vi "PH_Synchrolock_Watch.destructor.vi"(0 "i ref in":refnum<vi>, 5 "error in(no error)":errorcluster) -> (19 "error out":errorcluster)   [LabVIEW 2014, in "PH_Synchrolock_Watch.lvlib"]
doc: "This is the destructor of a class.\n\nLicense Agreement for this software:\n\nCopyright (C)\nGesellschaft für Schwerionenforschung, GSI\nPlanckstr. 1\n64291 Darmstadt\nGermany\n\nContact: D.Beck@gsi.de \n\nThis program is free software; you can redistribute it and/or modify it under the terms of the \nGNU General Public License as published by the Free Software Foundation; either version 2 of \nthe license, or (at your option) any later version.\n\nThis program is distributed in the hope that it will be useful, but WITHOUT ANY WARRANTY; \nwithout even the implied warranty of MERCHANTABILITY or FITNESS FOR A PARTICULAR PURPOSE. See the GNU General License for more details (http://www.gnu.org).\n\nGesellschaft für Schwerionenforschung, GSI\nPlanckstr. 1, 64291 Darmstadt, Germany\nFor all questions and ideas contact: M.Richter@gsi.de, H.Brand@gsi.de or D.Beck@gsi.de.\nLast update: 16-JUN-2004"
uses:
  PH_Synchrolock_Watch.lvlib
  PH_Devices/PH_TKTDS-30xx/PH_TKTDS-30xx.lvlib
  CS_Core/BaseProcess/BaseProcess.lvlib
  PH_Basics/PH_StatusHandler/PH_StatusHandler.lvlib
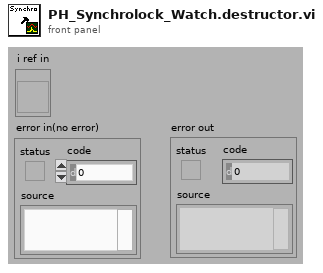
[diagram p1: front panel]
types:
  T1 = typedef "BaseProcess.lvlib/BaseProcess.i attribute.ctl" = cluster{"EventStatus":string, "EventError":i32, "PresetEvtWatchD":i32, "PresetPdcWatchD":i32, "EventTimeout":i32, "PeriodicInterval":i32, "Interface":string[], "Address":string[], "Special":string[], "PeriodicError":i32, "PeriodicStatus":string, "SuperProc":string, "Descriptors":T2[], "CaseRef":refnum<vi>, "PdcRef":refnum<vi>, "Thread Ref":refnum<vi>, "eventErrorID":i32, "eventStatusID":i32, "periodicErrorID":i32, "periodicStatusID":i32, "pdcCtrID":i32}
  T2 = typedef "BaseProcess.lvlib/BaseProcess.descriptor definition.ctl" = cluster{"selector":string, "descriptor":T3}
  T3 = typedef "BaseProcess.lvlib/BaseProcess.descriptor string definition.ctl" = string
  T4 = enum16{"SetAttribute", "GetAttribute", "CreateAttribute", "DestroyAttribute", "DestroyAllAtributes"}
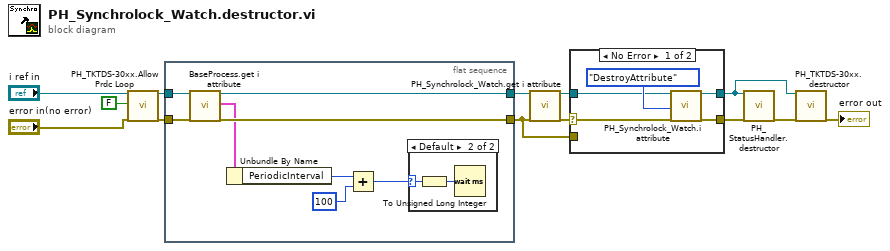
[diagram p0: block diagram]
diagram:
  n1 = call "PH_TKTDS-30xx.Allow Prdc Loop.vi"("i ref in"="i ref in", "Allow Prdc Loop?"=FALSE, "error in"="error in(no error)") -> ("i ref out"=w8:refnum<vi>, "error out"=w7:errorcluster)  [unwired: 15 in]
  n2 = flat-sequence {
    tunnel: w7 -> [w21]
    tunnel: [w20] -> w4
    tunnel: w8 -> [w19]
    tunnel: [w18] -> w6
    frame #0 {
      n3 = call "BaseProcess.get i attribute.vi"("i ref in"=w19, "error in (no error)"=w21) -> ("i ref out"=w18:refnum<vi>, "i attribute"=w17:T1, "error out"=w20:errorcluster)  [unwired: 15 in]
      n4 = Unbundle By Name(w17) -> ("PeriodicInterval"=w16:i32)
      n5 = Add(x=w16, y=100) -> (x+y=w14:i32)
      n6 = case shown="Default" w14 {
        selector: w14 -> [_ w23]
        frame -1 {
        }
        frame Default {
          n7 = To Unsigned Long Integer(number=w23) -> (unsigned 32bit integer=w22:u32)
          n8 = Wait (ms)(milliseconds to wait=w22) -> ()  [unwired: 1 out]
        }
      }
    }
  }
  n9 = call "PH_Synchrolock_Watch.get i attribute.vi"("i ref in"=w6, "error in (no error)"=w4) -> ("i ref out"=w11:refnum<vi>, "error out"=w5:errorcluster)  [unwired: 15 in, 1 out]
  n10 = case shown="No Error" w5 {
    selector: w5 -> [w24 _]
    tunnel: [w28 w29] -> w13
    tunnel: w11 -> [w26 w30]
    tunnel: [w25 w30] -> w1
    tunnel: w4 -> [_ w29]
    frame No Error {
      n11 = call "PH_Synchrolock_Watch.i attribute.vi"("VI Refnum"=w26, "Action"=T4."DestroyAttribute", "error in (no error)"=w24) -> ("VI Refnum out"=w25:refnum<vi>, "error out"=w28:errorcluster)  [unwired: 14 in, 1 out]
    }
    frame Error {
    }
  }
  n12 = call "PH_StatusHandler.destructor.vi"("i ref in"=w1, "error in(no error)"=w13) -> ("error out"=w2:errorcluster)  [unwired: 17 in]
  n13 = call "PH_TKTDS-30xx.destructor.vi"("i ref in"=w1, "error in(no error)"=w2) -> ("error out"=→"error out":errorcluster)  [unwired: 17 in]
